vi "Configure Functions.vi"(0 "instrument handle":refnum<k15>, 1 "Operand1 (Trace1)":i32(ring) items=["Trace1", "Trace2", "Trace3", "Trace4", "Trace5", "Trace6"], 2 "LogOffset":dbl, 5 "Trace":string="Trace1" caption="Trace (Trace1)", 7 "Destination (Trace1)":i32(ring) items=["Trace1", "Trace2", "Trace3", "Trace4", "Trace5", "Trace6"], 9 "Function (Off)":i32(ring) items=["Off", "Power Difference", "Power Sum", "Log Offset", "Log Difference"], 11 "error in (no error)":errorcluster {"code" format="%.0x"}, 12 "Operand2 (Trace1)":i32(ring) items=["Trace1", "Trace2", "Trace3", "Trace4", "Trace5", "Trace6"], 13 "LogDifferenceReference":dbl) -> (4 "instrument handle out":refnum<k15>, 15 "error out":errorcluster {"code" format="%.0x"})   [LabVIEW 2009, in "Keysight XSAn.lvlib"]
doc: "Turns on and configures trace math functions. Trace math functions perform mathematical operations between traces and, in some cases, user-specified offsets. When in a trace math function, the indicated function is performed during the sweep with the math function used in place of a detector. For some of the math modes some of the parameters are not relevant. For those modes, the parameters are ignored.\n\nSupported Models: M9290A, N8973B, N8974B, N8975B, N8976B, N9000A, N9000B, N9010A, N9010B, N9020A, N9020B, N9030A, N9030B, N9038A, N9040B, N9041B, SPN9003A, SPN9026A"
uses:
  <instrlib>/Keysight XSAn/Keysight XSAn.lvlib
  AgXSAn.dll
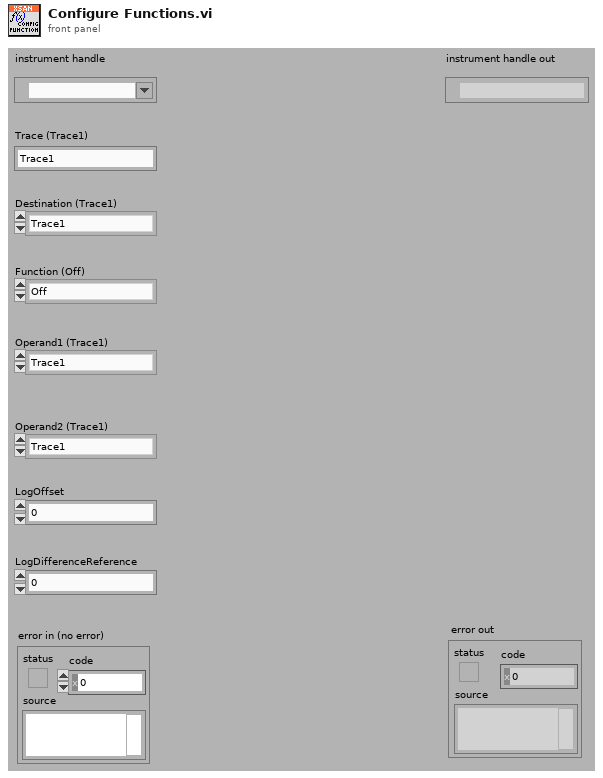
[diagram p1: front panel]
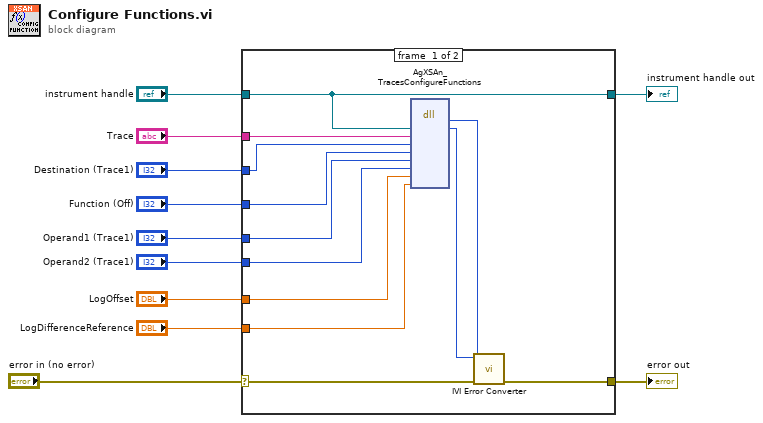
[diagram p0: block diagram]
diagram:
  n1 = case shown="No Error" "error in (no error)" {
    selector: "error in (no error)" -> [w21 w25]
    tunnel: [w20 w25] -> w11
    tunnel: "instrument handle" -> [w12 w24]
    tunnel: "Trace" -> [w19 _]
    tunnel: "Destination (Trace1)" -> [w18 _]
    tunnel: "Function (Off)" -> [w17 _]
    tunnel: "Operand1 (Trace1)" -> [w16 _]
    tunnel: "Operand2 (Trace1)" -> [w15 _]
    tunnel: "LogOffset" -> [w14 _]
    tunnel: "LogDifferenceReference" -> [w13 _]
    tunnel: [w12 w24] -> w1
    frame #0 {
      n2 = dll-call lib="AgXSAn**.dll" fn="AgXSAn_TracesConfigureFunctions"("Vi"=w12, "Trace"=w19, "Destination"=w18, "Function"=w17, "Operand1"=w16, "Operand2"=w15, "LogOffset"=w14, "LogDifferenceReference"=w13) -> (w22:i32, "Vi"=w23:u32)  [unwired: 10 in, 2 out]
      n3 = call <instrlib>:"IVI Error Converter.vi"("error in (no error)"=w21, "IVI error code (0)"=w22, "instrument handle"=w23) -> ("error out"=w20:errorcluster)  [unwired: 7 in, 1 out]
    }
    frame #1 {
    }
  }
  "error out" <- w11
  "instrument handle out" <- w1
